vi "Example Export.vi"() -> ()   [LabVIEW 2019]
doc: "Example VI to export a VI Snippet (*.png) programmatically.\n\nCreated by: Ryan Pacini"
uses:
  VI Snippet.lvlib
panel:
  in  "Selected GObjects Only? (F)":bool
  in  "VI Snippet Path (*.png)":path=path "C:/Projects/git/labview_snippet/src/Images/example.png"
  out "error out":errorcluster
  # "Export a VI Snippet (*.png) programmatically"
  # "(See Block Diagram for Instructions)"
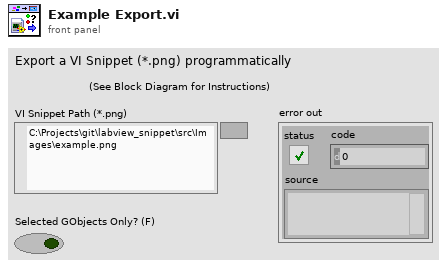
[diagram p1: front panel]
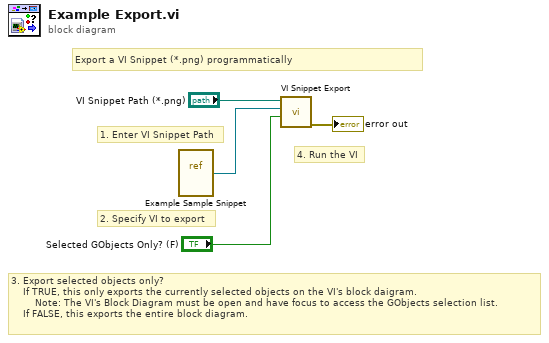
[diagram p0: block diagram]
diagram:
  # "3. Export selected objects only?\n    If TRUE, this only exports the currently selected objects on the VI's block daigram.\n        Note: The VI's Block Diagram must be open and have focus to access the GObjects selection list.\n    If FALSE, this exports the entire block diagram."
  # "2. Specify VI to export"
  # "4. Run the VI"
  # "1. Enter VI Snippet Path"
  # "Export a VI Snippet (*.png) programmatically"
  n1 = vi-ref "Example Sample Snippet.vi"() -> (w2:refnum<vi>)
  n2 = call "VI Snippet Export.vi"("Selected GObjects Only? (F)"="Selected GObjects Only? (F)", "VI Refnum"=w2, "VI Snippet Path (*.png)"="VI Snippet Path (*.png)") -> ("error out"=→"error out":errorcluster)  [unwired: 8 in]
